vi "例4.11-1 循环结构+条件结构.vi"() -> ()   [LabVIEW 2017]
panel:
  out "数组":i32[](array[numeric])
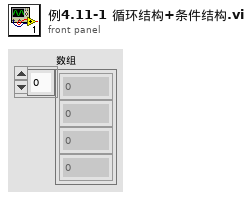
[diagram p1: front panel]
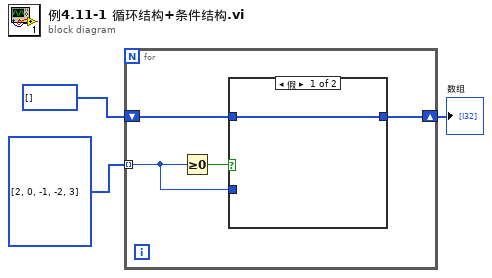
[diagram p0: block diagram]
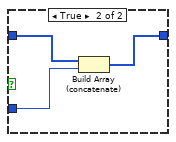
[diagram p2: hidden frame]
diagram:
  n1 = for {
    tunnel: i32[] [2, 0, -1, -2, 3] -> [w5] mode=indexing
    shift-right: [w7] -> w1
    shift-left: i32[] [] -> [w6]
    n2 = Greater Or Equal To 0?(x=w5) -> (x >= 0?=w4:bool)
    n3 = case shown="假" w4 {
      tunnel: [w8 w11] -> w7
      tunnel: w6 -> [w8 w10]
      tunnel: w5 -> [_ w9]
      frame False {
      }
      frame True {
        n4 = Build Array (concatenate)(w10, w9) -> (w11:i32[])
      }
    }
  }
  "数组" <- w1
